vi "Colonoscopy competition - Trajectory.vi"() -> (3 "Array":i32[][](array[numeric])=[[0, 0], [60, 60], [120, 60], [120, 120], [60, 120], [60, 60]])   [LabVIEW 2016]
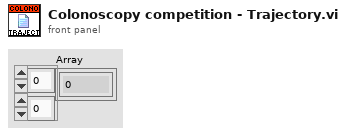
[diagram p1: front panel]
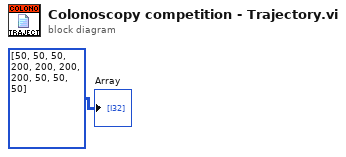
[diagram p0: block diagram]
diagram:
  "Array" <- i32[][] [[50, 50], [50, 200], [200, 200], [200, 50], [50, 50]]
